vi "OMV_UploadMainPY.vi"(9 "Script":string, 10 "Tx Buffer":string, 11 "VISA Refnum in":refnum<visa-resource-name>) -> (2 "Tx Buffer Out":string)   [LabVIEW 2016]
panel:
  out "read buffer":string
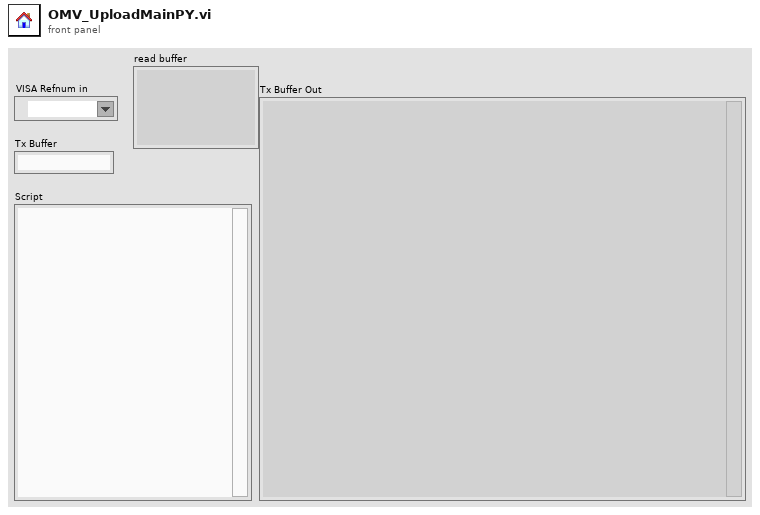
[diagram p1: front panel]
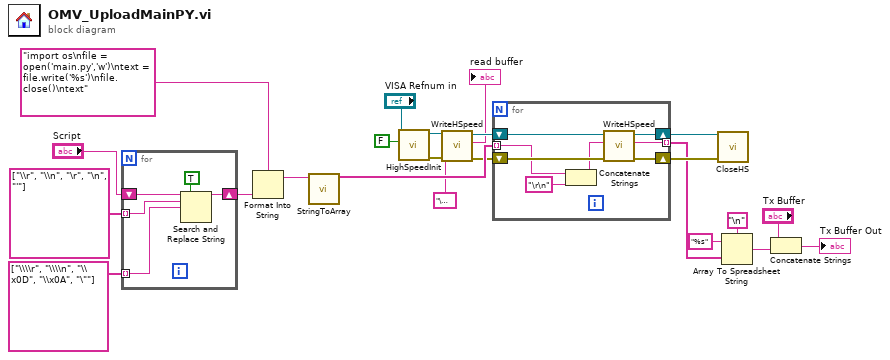
[diagram p0: block diagram]
diagram:
  n1 = for {
    shift-right: [w26] -> w20
    shift-left: "Script" -> [w28]
    tunnel: string[] ["\\r", "\\n", "\r", "\n", "'"] -> [w25] mode=indexing
    tunnel: string[] ["\\\\r", "\\\\n", "\\x0D", "\\x0A", "\""] -> [w24] mode=indexing
    n2 = Search and Replace String(replace all?=TRUE ("replace all? (F)"), input string=w28, search string=w25, replace string=w24) -> (result string=w26:string)  [unwired: 4 in, 3 out]
  }
  n3 = Format Into String(format string="import os\nfile = open('main.py','w')\ntext = file.write('%s')\nfile.close()\ntext" ("write buffer"), w20) -> (resulting string=w15:string)  [unwired: 2 in, 1 out]
  n4 = call "StringToArray.vi"("write buffer"=w15) -> ("Array"=w14:string[])  [unwired: 10 in]
  n5 = call "HighSpeedInit.vi"("Fast"=FALSE, "VISA Refnum in"="VISA Refnum in") -> ("error out"=w11:errorcluster, "VISA Refnum out"=w10:refnum<visa-resource-name>)  [unwired: 8 in]
  n6 = call "WriteHSpeed.vi"("error in"=w11, "write buffer"="\u0003", "VISA Refnum in"=w10) -> ("error out"=w7:errorcluster, "read buffer"=→"read buffer":string, "VISA Refnum out"=w8:refnum<visa-resource-name>)  [unwired: 6 in]
  n7 = for {
    shift-right: [w33] -> w13
    shift-left: w7 -> [w36]
    shift-right: [w34] -> w12
    shift-left: w8 -> [w35]
    tunnel: w14 -> [w30] mode=indexing
    tunnel: [w32] -> w3 mode=indexing
    n8 = Concatenate Strings(w30, "\r\n" ("write buffer")) -> (w29:string)
    n9 = call "WriteHSpeed.vi"("error in"=w36, "write buffer"=w29, "VISA Refnum in"=w35) -> ("error out"=w33:errorcluster, "read buffer"=w32:string, "VISA Refnum out"=w34:refnum<visa-resource-name>)  [unwired: 6 in]
  }
  n10 = call "CloseHS.vi"("error in (no error)"=w13, "VISA Refnum in"=w12) -> ()  [unwired: 10 in]
  n11 = Array To Spreadsheet String(delimiter (Tab)="\n", array=w3, 3:"%s" ("format string")) -> (spreadsheet string=w4:string)
  n12 = Concatenate Strings("Tx Buffer", w4) -> (→"Tx Buffer Out":string)
